vi "ex_SaveFileCheckName.vi"(4 "file exists?":bool, 5 "overwrite_mode_multi":T3(ring)=enum."overwrite & backup", 6 "multi_file":bool, 7 "overwrite_mode":T5(ring), 8 "error in (no error)":errorcluster, 9 "enable file ops":bool, 10 "file params in":T1={"delimiter"="\t", "origin time"=timestamp(0 s since 1904-01-01), "Flags"={"include col headings?"=TRUE, "x_columns"=0, "col headings always?"=TRUE, "time preference"=0, "hide col headings"=FALSE}, "Decimal Separator"=""} {"Flags"."time preference" items=["Absolute", "Relative"]; "Flags"."x_columns" items=["None", "One", "Multiple"]; "origin time" format="%<%X\n%x>T"}, 11 "file path":path) -> (0 "error out":errorcluster, 1 "function":T4(ring), 2 "file params out":T1={"delimiter"="\t", "origin time"=timestamp(0 s since 1904-01-01), "Flags"={"include col headings?"=TRUE, "x_columns"=0, "col headings always?"=TRUE, "time preference"=0, "hide col headings"=FALSE}, "Decimal Separator"=""} {"Flags"."time preference" items=["Absolute", "Relative"]; "Flags"."x_columns" items=["None", "One", "Multiple"]; "origin time" format="%<%X\n%x>T"}, 3 "file path out":path)   [LabVIEW 2017]
uses:
  <vilib>/express/express output/ExFileWriteBlock.llb/ex_WriteFileParams.ctl
  <vilib>/express/express input/ExFileReadBlock.llb/ex_ReadFileParams.ctl
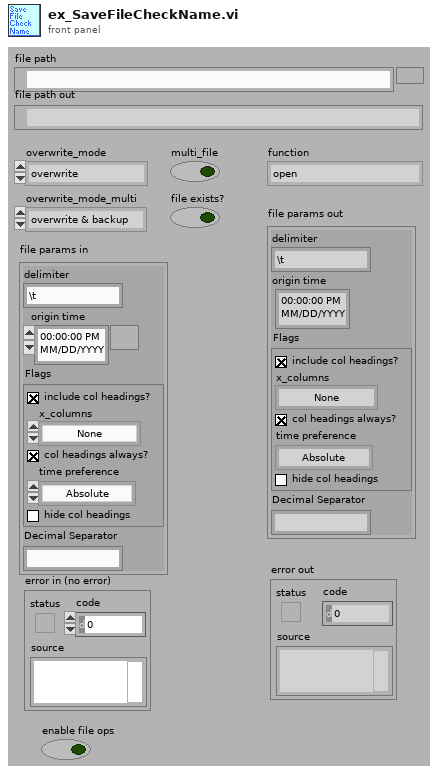
[diagram p1: front panel]
types:
  T1 = typedef "ex_WriteFileParams.ctl" = cluster{"delimiter":string, "origin time":timestamp, "Flags":T2, "Decimal Separator":string}
  T2 = typedef "ex_ReadFileParams.ctl" = cluster{"include col headings?":bool, "x_columns":u16, "col headings always?":bool, "time preference":u16, "hide col headings":bool}
  T3 = enum16{"overwrite", "overwrite & backup", "next avail"}
  T4 = enum16{"open", "open or create", "create or replace", "create", "open (read only)"}
  T5 = enum16{"overwrite", "overwrite & backup", "append", "next avail"}
  T6 = typedef "ex_FileReference.ctl" = cluster{"file ref":refnum<file>, "file size (bytes:0)":i32, "read pointer (bytes:0)":i32, "chunk size (bytes:65000)":i32}
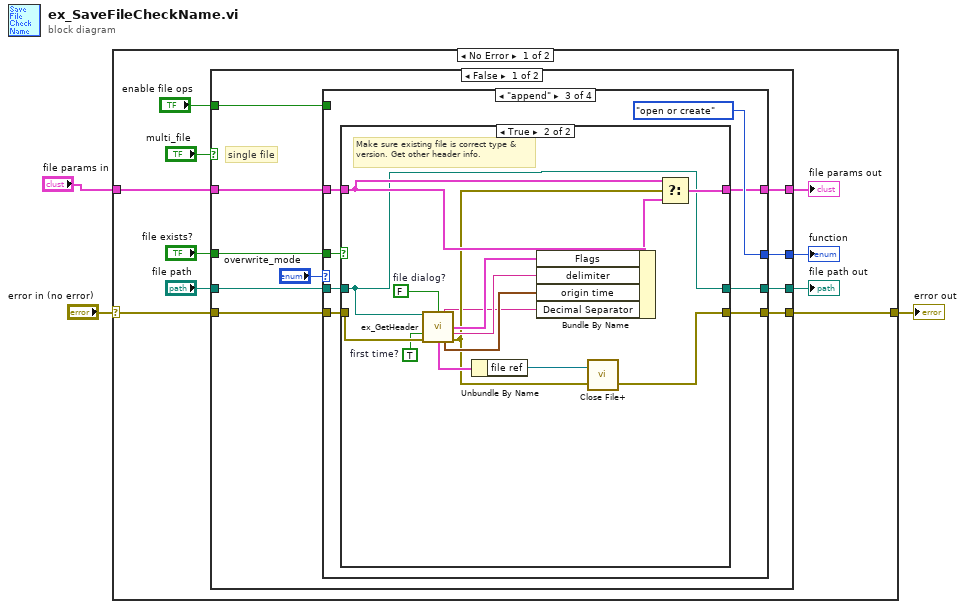
[diagram p0: block diagram]
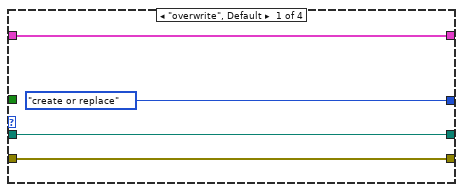
[diagram p2: hidden frame]
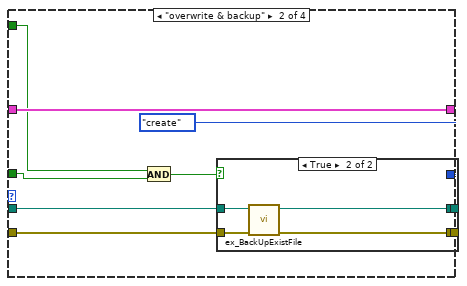
[diagram p3: hidden frame]
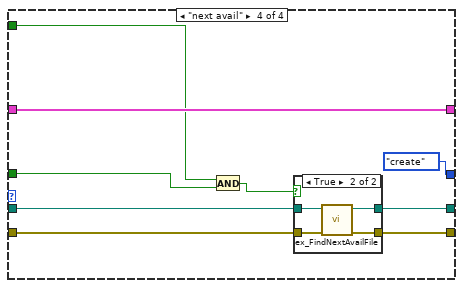
[diagram p6: hidden frame]
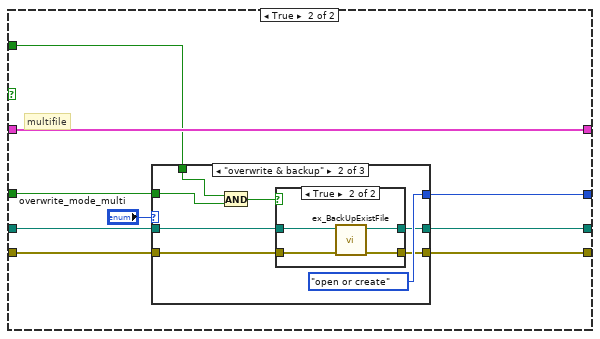
[diagram p8: hidden frame]
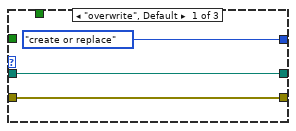
[diagram p9: hidden frame]
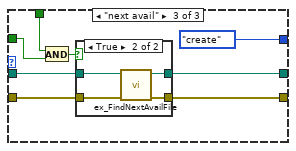
[diagram p11: hidden frame]
diagram:
  n1 = case shown="No Error" "error in (no error)" {
    selector: "error in (no error)" -> [w7 w124]
    tunnel: [w9 w124] -> w3
    tunnel: "file params in" -> [w4 _]
    frame No Error {
      n2 = case shown="False" "multi_file" {
        tunnel: [w22 w91] -> w13
        tunnel: "file path" -> [w17 w90]
        tunnel: [w19 w88] -> w10
        tunnel: [w18 w87] -> w9
        tunnel: "file exists?" -> [w21 w86]
        tunnel: w7 -> [w20 w89]
        tunnel: [w15 w85] -> w6
        tunnel: w4 -> [w16 w85]
        tunnel: "enable file ops" -> [w14 w84]
        frame False {
          # "single file"
          n3 = case shown="\"append\"" "overwrite_mode" {
            tunnel: [T4."create or replace" ("function (open:0)") T4."create" ("function (open:0)") T4."open or create" ("function (open:0)") T4."create" ("function (open:0)")] -> w22
            tunnel: w21 -> [_ w29 w48 w70]
            tunnel: w17 -> [w26 w33 w44 w76]
            tunnel: w20 -> [w25 w32 w49 w73]
            tunnel: [w26 w35 w43 w74] -> w19
            tunnel: [w25 w34 w47 w75] -> w18
            tunnel: [w24 w31 w46 w72] -> w15
            tunnel: w16 -> [w24 w31 w45 w72]
            tunnel: w14 -> [_ w28 _ w69]
            frame "overwrite", Default {
            }
            frame "overwrite & backup" {
              n4 = And(x=w28, y=w29) -> (x .and. y?=w30:bool)
              n5 = case shown="True" w30 {
                tunnel: w33 -> [w37 w40]
                tunnel: w32 -> [w38 w39]
                tunnel: [w37 w42] -> w35
                tunnel: [w38 w41] -> w34
                frame False {
                  # "File doesn't exist-- do nothing"
                }
                frame True {
                  n6 = call <vilib>:"ex_BackUpExistFile.vi"("error in"=w39, "file path"=w40) -> ("error out"=w41:errorcluster, "dup file path"=w42:path)  [unwired: 8 out]
                }
              }
            }
            frame "append" {
              n7 = case shown="True" w48 {
                tunnel: w49 -> [w52 w68]
                tunnel: w44 -> [w51 w58]
                tunnel: [w52 w57] -> w47
                tunnel: [w53 w65] -> w46
                tunnel: w45 -> [w53 w64]
                tunnel: [w51 w58] -> w43
                frame False {
                }
                frame True {
                  w66 = TRUE  # first time?
                  w67 = FALSE  # file dialog?
                  # "Make sure existing file is correct type & version. Get other header info."
                  n8 = call <vilib>:"ex_GetHeader.vi"("file path"=w58, "file dialog?"=w67, "first_time?"=w66, "error in (no error)"=w68) -> ("Decimal Separator"=w54:string, "file_params"=w61:T2, "delimiter"=w59:string, "file refs out"=w60:T6, "origin timestamp"=w62:timestamp, "error out"=w56:errorcluster)  [unwired: 2 in, 4 out]
                  n9 = Unbundle By Name(w60) -> ("file ref"=w55:refnum<file>)
                  n10 = Bundle By Name(cluster=w64, "Flags"=w61, "delimiter"=w59, "origin time"=w62, "Decimal Separator"=w54) -> (w63:T1)
                  n11 = call <vilib>:"Close File+.vi"("error in (no error)"=w56, "refnum"=w55) -> ("error out"=w57:errorcluster)  [unwired: 5 out]
                  n12 = Select(t=w64, s=w56, f=w63) -> (s? t:f=w65:T1)
                }
              }
            }
            frame "next avail" {
              n13 = And(x=w69, y=w70) -> (x .and. y?=w71:bool)
              n14 = case shown="True" w71 {
                tunnel: w76 -> [w79 w83]
                tunnel: [w78 w82] -> w75
                tunnel: [w79 w81] -> w74
                tunnel: w73 -> [w78 w80]
                frame False {
                }
                frame True {
                  n15 = call <vilib>:"ex_FindNextAvailFile.vi"("error in"=w80, "desired file path"=w83) -> ("error out"=w82:errorcluster, "next avail file path"=w81:path)  [unwired: 8 out]
                }
              }
            }
          }
        }
        frame True {
          # "multifile"
          n16 = case shown="\"overwrite & backup\"" "overwrite_mode_multi" {
            tunnel: [T4."create or replace" ("function (open:0)") T4."open or create" ("function (open:0)") T4."create" ("function (open:0)")] -> w91
            tunnel: w90 -> [w94 w102 w114]
            tunnel: w89 -> [w93 w101 w113]
            tunnel: [w94 w100 w116] -> w88
            tunnel: [w93 w99 w115] -> w87
            tunnel: w86 -> [_ w97 w111]
            tunnel: w84 -> [_ w96 w110]
            frame "overwrite", Default {
            }
            frame "overwrite & backup" {
              n17 = And(x=w96, y=w97) -> (x .and. y?=w98:bool)
              n18 = case shown="True" w98 {
                tunnel: w102 -> [w104 w107]
                tunnel: w101 -> [w105 w106]
                tunnel: [w104 w109] -> w100
                tunnel: [w105 w108] -> w99
                frame False {
                  # "File doesn't exist-- do nothing"
                }
                frame True {
                  n19 = call <vilib>:"ex_BackUpExistFile.vi"("error in"=w106, "file path"=w107) -> ("error out"=w108:errorcluster, "dup file path"=w109:path)  [unwired: 8 out]
                }
              }
            }
            frame "next avail" {
              n20 = And(x=w110, y=w111) -> (x .and. y?=w112:bool)
              n21 = case shown="True" w112 {
                tunnel: w114 -> [w119 w123]
                tunnel: [w118 w122] -> w115
                tunnel: [w119 w121] -> w116
                tunnel: w113 -> [w118 w120]
                frame False {
                }
                frame True {
                  n22 = call <vilib>:"ex_FindNextAvailFile.vi"("error in"=w120, "desired file path"=w123) -> ("error out"=w122:errorcluster, "next avail file path"=w121:path)  [unwired: 8 out]
                }
              }
            }
          }
        }
      }
      "function" <- w13
      "file path out" <- w10
      "file params out" <- w6
    }
    frame Error {
    }
  }
  "error out" <- w3
